vi "FTW-Actor-Initialize.vi"(0 "FTW Actor Instance Type":refnum<class "FTW-Actor-Instance.lvclass">, 5 "Initialization Job Sequence":string, 7 "Actor Instance Configuration":string, 11 "error in":errorcluster) -> (4 "FTW Actor Instance":refnum<class "FTW-Actor-Instance.lvclass">, 6 "Incoming Request":refnum<event-registration>, 15 "error out":errorcluster)   [LabVIEW 2013, in "FTW-Actor-Instance.lvclass"]
uses:
  FTW-Actor-Instance.lvclass
  message/FTW-Message.lvclass
  socket/FTW-Socket-Type.ctl
  socket/FTW-Socket.lvclass
  FTW-Actor-Instance.lvclass/FTW-Actor-Instance.ctl
  error/FTW-ERR-ThrowError.vi
  error/FTW-ERR-NoErrorConstant.vi
  reflection/FTW-Reflection-Type.vi
  json/lib/FTW-JSON-Core-LibraryFilepath.vi
  json/lib/FTW-JSON-Core-GetFlattenedValue.vi
  json/lib/FTW-JSON-Core-LibraryError.vi
  error/FTW-ERR-CallChain.vi
  string/FTW-STR-ReplaceWhitespace.vi
  json/FTW-JSON-Deserialize/FTW-JSON-Deserialize.xnode
  scheduler/FTW-Scheduler.lvclass
  logger/FTW-Logger.lvclass
  router/FTW-Router.lvclass
panel:
  # "Inputs"
  # "Outputs"
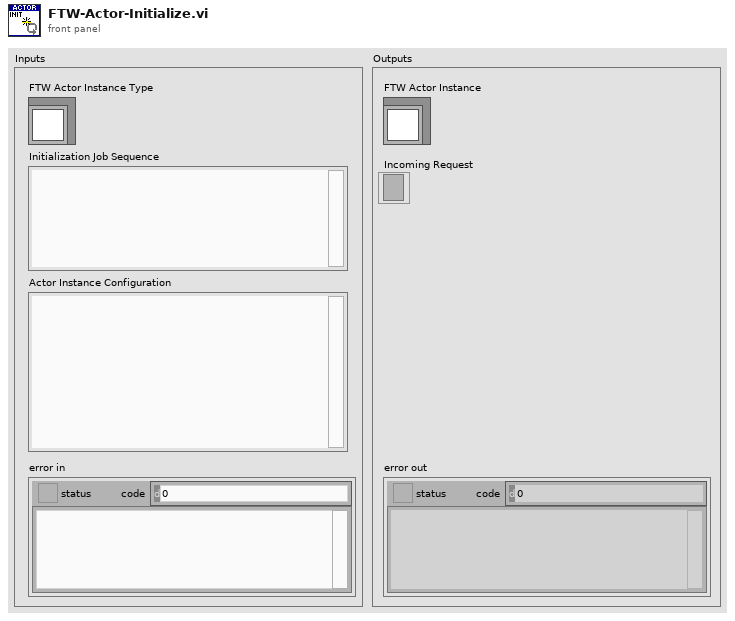
[diagram p1: front panel]
types:
  T1 = typedef "FTW-Socket.lvclass/FTW-Socket-Type.ctl" = enum32{"Server", "Client", "Publisher", "Subscriber", "Pipeline Producer", "Pipeline Consumer", "Surveyor", "Respondent", "Exclusive Pair", "Bus"}
  T2 = cluster{"Identity":string, "InboxAddress":string, "PublisherAddress":string, "LoggerAddress":string, "LauncherAddress":string, "DebugEnableInboxLogging":bool, "DebugEnableJobLogging":bool, "LaunchTimeout":i32}
  T3 = cluster{"Inbox Address":string, "Actual Endpoint Address":string}
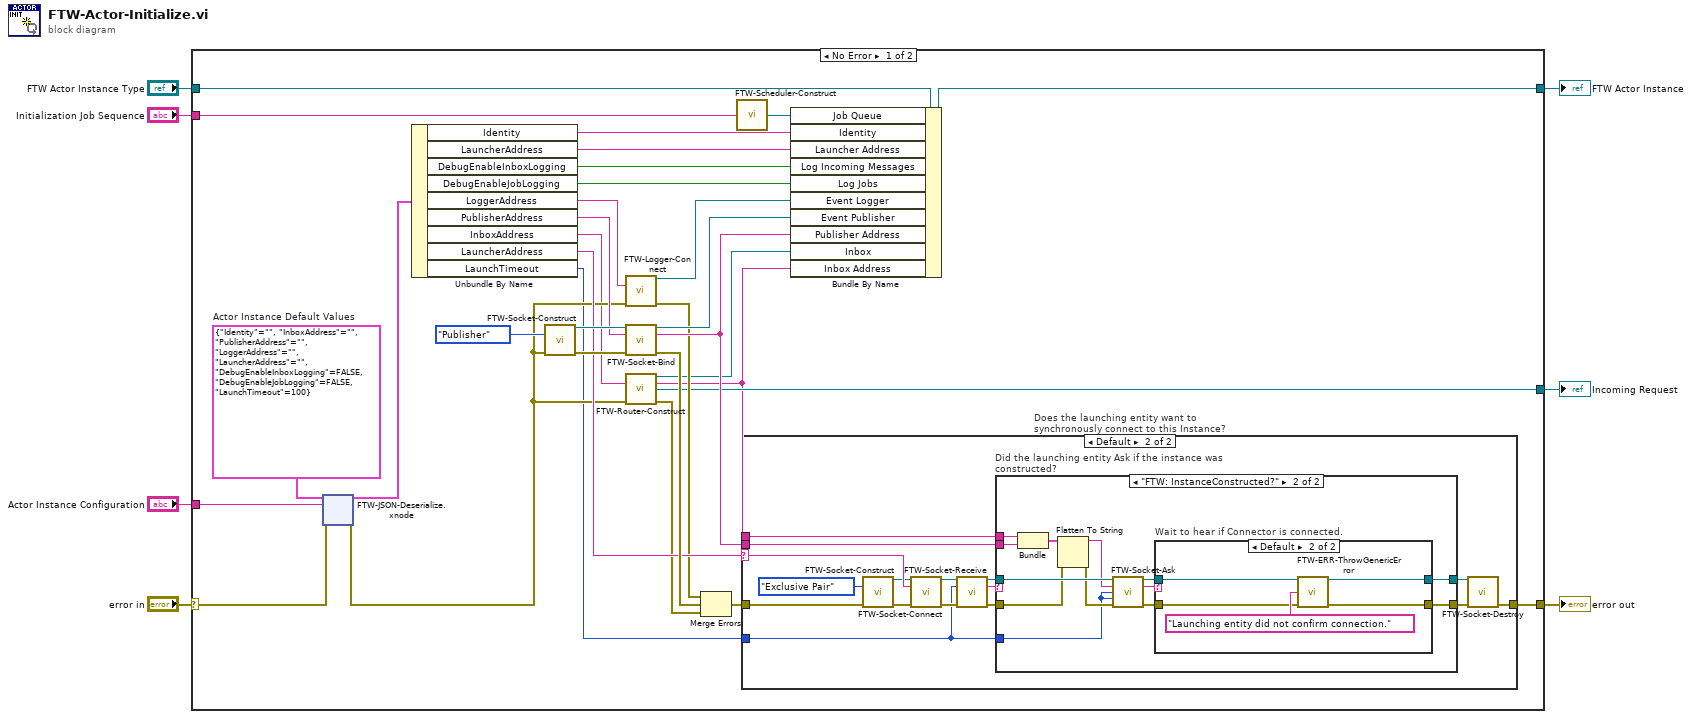
[diagram p0: block diagram]
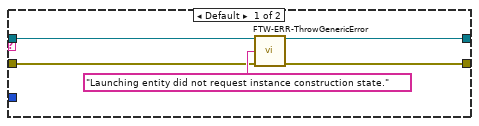
[diagram p3: hidden frame]
diagram:
  n1 = case shown="No Error" "error in" {
    selector: "error in" -> [w30 w115]
    tunnel: "FTW Actor Instance Type" -> [w37 w114]
    tunnel: [w36 w115] -> w6
    tunnel: [w10 _] -> w5
    tunnel: "Initialization Job Sequence" -> [w35 _]
    tunnel: [w34 w114] -> w3
    tunnel: "Actor Instance Configuration" -> [w33 _]
    frame No Error {
      w32 = T2 {"Identity"="", "InboxAddress"="", "PublisherAddress"="", "LoggerAddress"="", "LauncherAddress"="", "DebugEnableInboxLogging"=FALSE, "DebugEnableJobLogging"=FALSE, "LaunchTimeout"=100}  # Actor Instance Default Values
      n2 = xnode "FTW-JSON-Deserialize.xnode"("Type and Defaults"=w32, "JSON String"=w33, "error in"=w30) -> ("Values"=w31:T2, "error out"=w14:errorcluster)
      n3 = Unbundle By Name(w31) -> ("Identity"=w29:string, "LauncherAddress"=w28:string, "DebugEnableInboxLogging"=w20:bool, "DebugEnableJobLogging"=w19:bool, "LoggerAddress"=w17:string, "PublisherAddress"=w22:string, "InboxAddress"=w13:string, "LauncherAddress"=w18:string, "LaunchTimeout"=w8:i32)
      n4 = call "FTW-Socket-Construct.vi"("Socket Topology"=FTW-Socket-Type."Publisher", "error in"=w14) -> ("FTW Socket"=w26:refnum<class "FTW-Socket.lvclass">, "error out"=w25:errorcluster)  [unwired: 12 in]
      n5 = call "FTW-Logger-Connect.vi"("Logger Address"=w17, "error in"=w14) -> ("FTW Logger Connector"=w15:refnum<class "FTW-Logger.lvclass">, "error out"=w16:errorcluster)  [unwired: 12 in]
      n6 = call-dynamic "FTW-Socket-Bind.vi"("FTW Endpoint"=w26, "Remote Endpoint Address"=w22, "error in"=w25) -> ("FTW Endpoint out"=w24:refnum<class "FTW-Socket.lvclass">, "Actual Endpoint Address"=w23:string, "error out"=w39:errorcluster)  [unwired: 10 in]
      n7 = call "FTW-Router-Construct.vi"("Incoming Message Router Address"=w13, "error in"=w14) -> ("FTW Router"=w11:refnum<class "FTW-Router.lvclass">, "Inbox Address"=w9:string, "Incoming Message"=w10:refnum<event-registration>, "error out"=w12:errorcluster)  [unwired: 10 in]
      n8 = Merge Errors(w16, w39, w12) -> (w21:errorcluster)
      n9 = call "FTW-Scheduler-Construct.vi"("Initial Job Sequence"=w35) -> ("FTW Job Scheduler"=w38:refnum<class "FTW-Scheduler.lvclass">)
      n10 = case "Does the launching entity want to synchronously connect to this Instance?" shown="Default" w18 {
        selector: w18 -> [_ w82]
        tunnel: w21 -> [w74 w81]
        tunnel: w9 -> [_ w90]
        tunnel: [w74 w86] -> w36
        tunnel: w23 -> [_ w84]
        tunnel: w8 -> [_ w76]
        frame "" {
        }
        frame Default {
          n11 = call "FTW-Socket-Construct.vi"("Socket Topology"=FTW-Socket-Type."Exclusive Pair" ("Socket Type"), "error in"=w81) -> ("FTW Socket"=w80:refnum<class "FTW-Socket.lvclass">, "error out"=w79:errorcluster)  [unwired: 12 in]
          n12 = call "FTW-Socket-Connect.vi"("FTW Socket"=w80, "Remote Address"=w82, "error in"=w79) -> ("FTW Socket out"=w78:refnum<class "FTW-Socket.lvclass">, "error out"=w77:errorcluster)  [unwired: 11 in]
          n13 = call "FTW-Socket-Receive.vi"("FTW Socket"=w78, "Timeout"=w76, "error in"=w77) -> ("FTW Socket out"=w88:refnum<class "FTW-Socket.lvclass">, "Message"=w75:string, "error out"=w89:errorcluster)  [unwired: 9 in, 1 out]
          n14 = case "Did the launching entity Ask if the instance was constructed?" shown="\"FTW: InstanceConstructed?\"" w75 {
            tunnel: w90 -> [_ w102]
            tunnel: w89 -> [w91 w99]
            tunnel: w88 -> [w92 w107]
            tunnel: [w94 w104] -> w85
            tunnel: [w92 w103] -> w87
            tunnel: w84 -> [_ w101]
            tunnel: w76 -> [_ w96]
            frame Default {
              n15 = call "FTW-ERR-ThrowGenericError.vi"("Error Message"="Launching entity did not request instance construction state.", "error in"=w91) -> ("error out"=w94:errorcluster)  [unwired: 13 in]
            }
            frame "FTW: InstanceConstructed?" {
              n16 = Bundle("Inbox Address"=w102, "Actual Endpoint Address"=w101) -> (w100:T3)  [unwired: 1 in]
              n17 = Flatten To String(anything=w100, error in (no error)=w99) -> (data string=w97:string, error out=w98:errorcluster)  [unwired: 2 in, 1 out]
              n18 = call "FTW-Socket-Ask.vi"("FTW Socket"=w107, "Request"=w97, "Receive Timeout"=w96, "Send Timeout"=w96, "error in"=w98) -> ("FTW Socket out"=w106:refnum<class "FTW-Socket.lvclass">, "Response"=w95:string, "error out"=w105:errorcluster)  [unwired: 7 in, 1 out]
              n19 = case "Wait to hear if Connector is connected." shown="Default" w95 {
                tunnel: w106 -> [w109 w110]
                tunnel: w105 -> [w108 w112]
                tunnel: [w108 w111] -> w104
                tunnel: [w109 w110] -> w103
                frame "FTW: Connected!" {
                  # "All is good!"
                }
                frame Default {
                  n20 = call "FTW-ERR-ThrowGenericError.vi"("Error Message"="Launching entity did not confirm connection.", "error in"=w112) -> ("error out"=w111:errorcluster)  [unwired: 13 in]
                }
              }
            }
          }
          n21 = call-dynamic "FTW-Socket-Destroy.vi"("FTW Socket"=w87, "error in"=w85) -> ("error out"=w86:errorcluster)  [unwired: 13 in]
        }
      }
      n22 = Bundle By Name(cluster=w37, "Job Queue"=w38, "Identity"=w29, "Launcher Address"=w28, "Log Incoming Messages"=w20, "Log Jobs"=w19, "Event Logger"=w15, "Event Publisher"=w24, "Publisher Address"=w23, "Inbox"=w11, "Inbox Address"=w9) -> (w34:refnum<class "FTW-Actor-Instance.lvclass">)
    }
    frame Error {
    }
  }
  "FTW Actor Instance" <- w3
  "error out" <- w6
  "Incoming Request" <- w5
